vi "write_cmd_to_dynamixels.vi"(8 "Dynamixel Setpoint In (deg)":dbl, 9 "Dynamixel Cycle Number":i32, 10 "Motor ID":u8=2, 11 "VISA resource name":refnum<visa-resource-name>) -> (0 "Error out":errorcluster, 3 "Written value":dbl)   [LabVIEW 2013]
doc: "Because the Dynamixel is (theoretically) a 0-360 deg position controlled motor, we will need to only command 0-360 values, and keep track of the loop counts to find out where the motor really is. This really needs to be tested with the actual Dynamixels. When we aren't in the correct 0-360 degree range, this VI will drive the motor in wheel mode in the right direction, then will use position mode to set the motor.\n\nEric Schneider, March 2014"
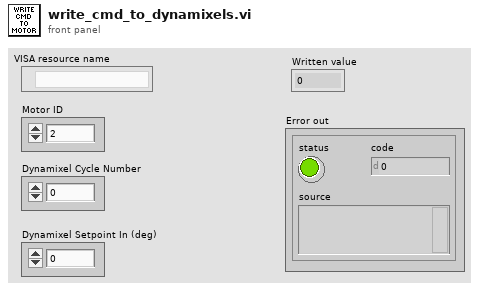
[diagram p1: front panel]
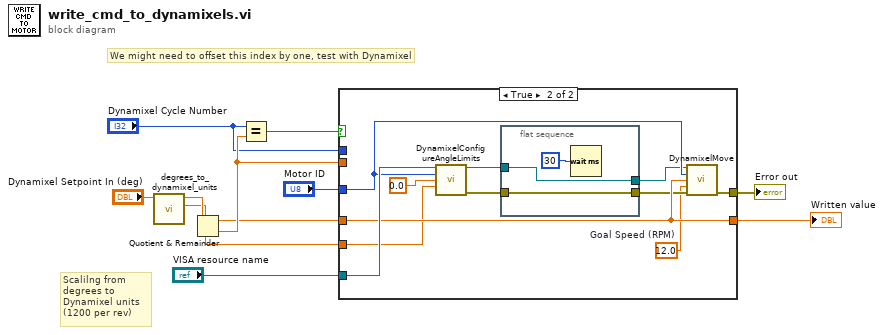
[diagram p0: block diagram]
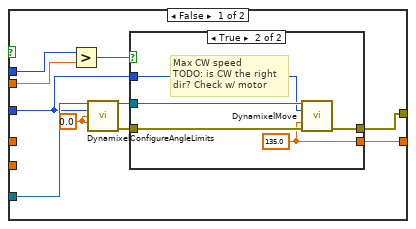
[diagram p2: hidden frame]
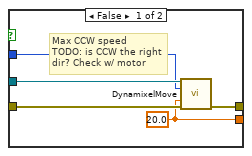
[diagram p3: hidden frame]
diagram:
  # "Scalilng from degrees to Dynamixel units (1200 per rev)"
  # "We might need to offset this index by one, test with Dynamixel"
  n1 = call "degrees_to_dynamixel_units.vi"("Degree Input"="Dynamixel Setpoint In (deg)") -> ("Dynamixel units/cycle"=w1:dbl, "Dynamixel units"=w5:dbl)  [unwired: 9 in]
  n2 = Quotient & Remainder(x=w5, y=w1) -> (x-y*floor(x/y)=w9:dbl, floor(x/y)=w10:dbl)
  n3 = Equal?(x="Dynamixel Cycle Number", y=w10) -> (x = y?=w11:bool)
  n4 = case shown="True" w11 {
    tunnel: w9 -> [_ w38]
    tunnel: "Dynamixel Cycle Number" -> [w21 _]
    tunnel: w10 -> [w20 _]
    tunnel: "VISA resource name" -> [w17 w41]
    tunnel: "Motor ID" -> [w13 w40]
    tunnel: [w18 w42] -> w6
    tunnel: [w12 w38] -> w3
    tunnel: w1 -> [_ w33]
    frame False {
      w14 = 0.0 ("Clockwise Angle Limit (0 deg)")
      n5 = Greater?(x=w21, y=w20) -> (0:w19:bool)
      n6 = call "DynamixelConfigureAngleLimits.vi"("VISA resource name"=w17, "Motor ID (0)"=w13, "Clockwise Angle Limit (0 deg)"=w14, "Counter-Clockwise Angle Limit (300 deg)"=w14) -> ("VISA resource name out"=w16:refnum<visa-resource-name>, "error out"=w15:errorcluster)  [unwired: 10 in]
      n7 = case shown="True" w19 {
        tunnel: w16 -> [w24 w31]
        tunnel: w13 -> [w23 w30]
        tunnel: w15 -> [w25 w29]
        tunnel: [w26 w28] -> w18
        tunnel: [w22 w27] -> w12
        frame False {
          w22 = 20.0 ("Goal Speed (RPM)")
          # "Max CCW speed\nTODO: is CCW the right dir? Check w/ motor"
          n8 = call "DynamixelMove.vi"("VISA resource name"=w24, "Motor ID (0)"=w23, "Goal Speed (RPM)"=w22, "error in (no error)"=w25) -> ("error out"=w26:errorcluster)  [unwired: 10 in, 1 out]
        }
        frame True {
          w27 = 135.0 ("Goal Speed (RPM)")
          # "Max CW speed\nTODO: is CW the right dir? Check w/ motor"
          n9 = call "DynamixelMove.vi"("VISA resource name"=w31, "Motor ID (0)"=w30, "Goal Speed (RPM)"=w27, "error in (no error)"=w29) -> ("error out"=w28:errorcluster)  [unwired: 10 in, 1 out]
        }
      }
    }
    frame True {
      w32 = 12.0  # Goal Speed (RPM)
      n10 = call "DynamixelConfigureAngleLimits.vi"("VISA resource name"=w41, "Motor ID (0)"=w40, "Clockwise Angle Limit (0 deg)"=0.0, "Counter-Clockwise Angle Limit (300 deg)"=w33) -> ("VISA resource name out"=w34:refnum<visa-resource-name>, "error out"=w37:errorcluster)  [unwired: 10 in]
      n11 = flat-sequence {
        tunnel: [w45] -> w36
        tunnel: w37 -> [w45]
        tunnel: [w44] -> w35
        tunnel: w34 -> [w44]
        frame #0 {
          n12 = Wait (ms)(milliseconds to wait=u32 30) -> ()  [unwired: 1 out]
        }
      }
      n13 = call "DynamixelMove.vi"("VISA resource name"=w35, "Motor ID (0)"=w40, "Goal Position (150 deg)"=w38, "Goal Speed (RPM)"=w32, "error in (no error)"=w36) -> ("error out"=w42:errorcluster)  [unwired: 9 in, 1 out]
    }
  }
  "Error out" <- w6
  "Written value" <- w3
